vi "Next Point.vi"(10 "Grid In":i64[][](graph), 11 "Point":cluster{"X":i32, "Y":i32}) -> (3 "Point out":cluster{"X":i32, "Y":i32})   [LabVIEW 2021]
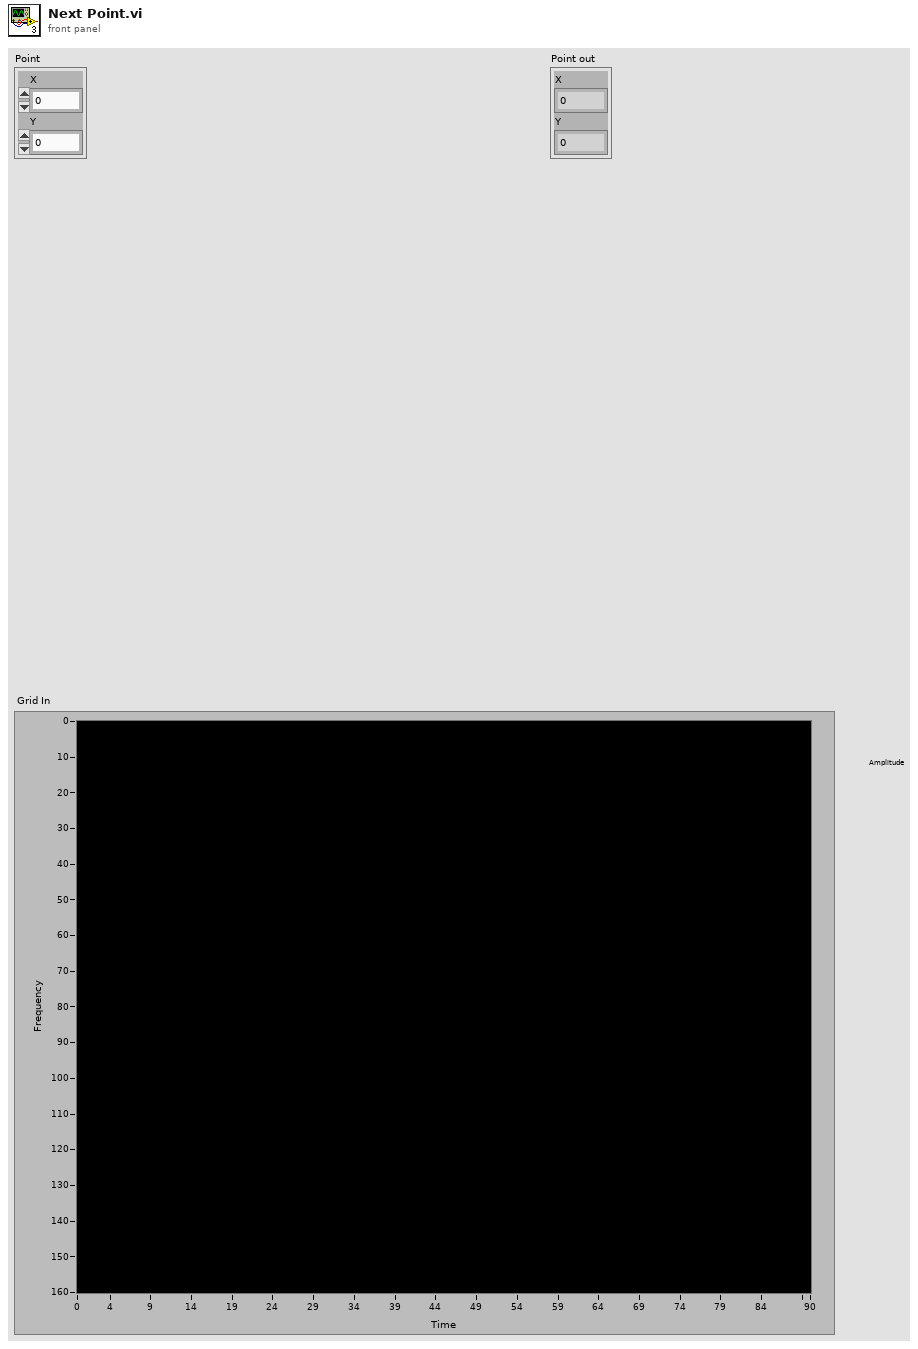
[diagram p1: front panel]
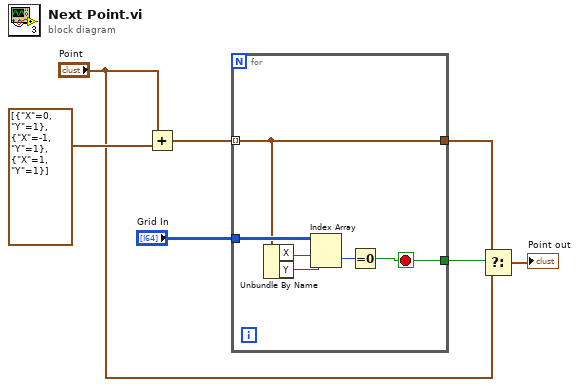
[diagram p0: block diagram]
diagram:
  n1 = Add(x="Point", y=cluster{"X":i32, "Y":i32}[] [{"X"=0, "Y"=1}, {"X"=-1, "Y"=1}, {"X"=1, "Y"=1}]) -> (x+y=w6:cluster{"X":i32, "Y":i32}[])
  n2 = for {
    tunnel: w6 -> [w9] mode=indexing
    tunnel: "Grid In" -> [w13]
    tunnel: [w9] -> w3
    tunnel: [w8] -> w4
    stop <- w8 stop-if-true
    n3 = Unbundle By Name(w9) -> ("X"=w12:i32, "Y"=w11:i32)
    n4 = Index Array(array=w13, index (row)=w12, index (col)=w11) -> (element=w10:i64)
    n5 = Equal To 0?(x=w10) -> (x = 0?=w8:bool)
  }
  n6 = Select(t=w3, s=w4, f="Point") -> (s? t:f=→"Point out":cluster{"X":i32, "Y":i32})
